vi "Pass If Equal String.vi"(8 "error in (no error)":errorcluster, 9 "actual":string, 10 "expected":string, 11 "TestCase in":refnum<class "TestCase.lvclass">) -> (0 "error out":errorcluster, 3 "TestCase out":refnum<class "TestCase.lvclass">)   [LabVIEW 2015, in "VITAC.lvlib"]
uses:
  VITAC.lvlib
  <vilib>/addons/_JKI Toolkits/VI Tester/TestCase.llb/TestCase.lvclass
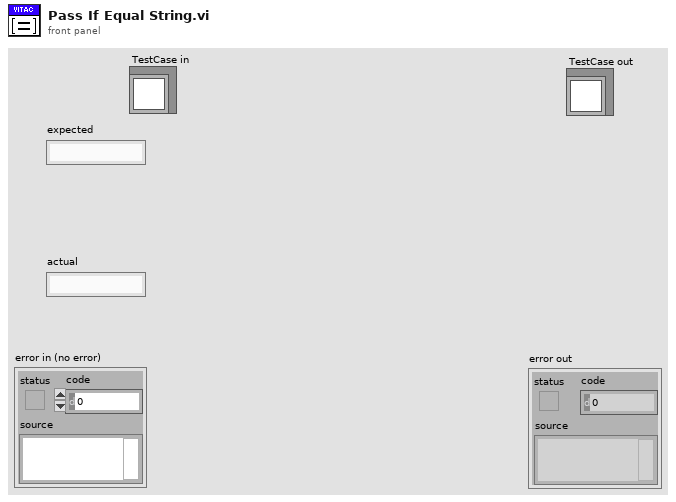
[diagram p1: front panel]
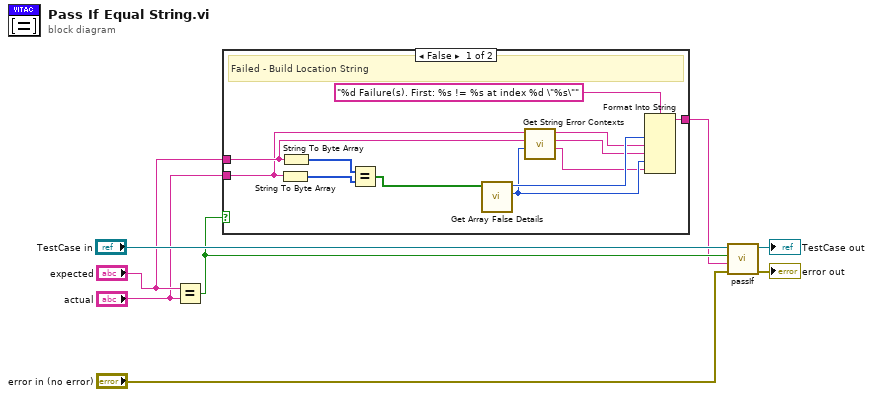
[diagram p0: block diagram]
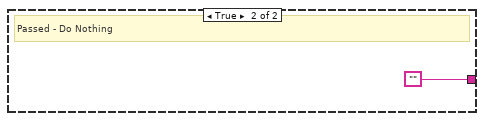
[diagram p2: hidden frame]
diagram:
  n1 = Equal?(x="expected", y="actual") -> (x = y?=w4:bool)
  n2 = case shown="False" w4 {
    tunnel: "expected" -> [w12 _]
    tunnel: "actual" -> [w11 _]
    tunnel: [w17 ""] -> w1
    frame False {
      # "Failed - Build Location String"
      n3 = String To Byte Array(string=w11) -> (unsigned byte array=w15:u8[])
      n4 = String To Byte Array(string=w12) -> (unsigned byte array=w16:u8[])
      n5 = Equal?(x=w16, y=w15) -> (x = y?=w14:bool[])
      n6 = call "Get Array False Details.vi"("Array"=w14) -> ("First False"=w10:i32, "Count"=w19:i16)  [unwired: 9 in]
      n7 = call "Get String Error Contexts.vi"("index of error"=w10, "expected string"=w12, "actual string"=w11) -> ("Actual Context"=w9:string, "expected char"=w18:string, "actual char"=w13:string)  [unwired: 6 in]
      n8 = Format Into String(format string="%d Failure(s). First: %s != %s at index %d \"%s\"", w19, w13, w18, w10, w9) -> (resulting string=w17:string)  [unwired: 2 in, 1 out]
    }
    frame True {
      # "Passed - Do Nothing"
    }
  }
  n9 = call-dynamic "passIf.vi"("error in (no error)"="error in (no error)", "message (\"\")"=w1, "pass"=w4, "TestCase in"="TestCase in") -> ("error out"=→"error out":errorcluster, "TestCase out"=→"TestCase out":refnum<class "TestCase.lvclass">)  [unwired: 6 in]
